vi "Module ID.vi"(11 "Historian Logger in":refnum<class "Historian Logger.lvclass">) -> (2 "Module ID":string)   [LabVIEW 2020, in "VolatusHistorian.lvlib" / "Historian Logger.lvclass"]
uses:
  Historian Logger.lvclass
  Historian Logger.lvclass/Historian Logger.ctl
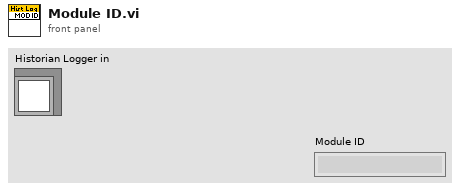
[diagram p1: front panel]
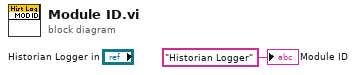
[diagram p0: block diagram]
diagram:
  "Module ID" <- "Historian Logger" ("Module ID")
